vi "Move to End.vi"   [LabVIEW 2017, in "Drivers.lvlib" / "ASI TG-1000.lvlib"]
uses:
  ASI TG-1000.lvlib
  Public/Utility/Axis Name.ctl
types:
  T1 = typedef "Drivers.lvlib/ASI TG-1000.lvlib/Axis Name.ctl" = enum8{"undefined", "A", "B", "C", "D", "E", "F", "G", "H", "I", "J", "K", "L", "M", "N", "O", "P", "Q", "R", "S", "T", "U", "V", "W", "X", "Y", "Z"}
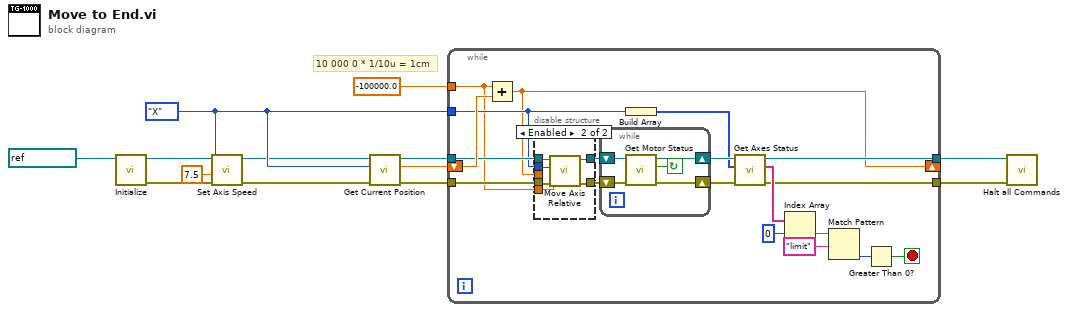
[diagram p0: block diagram]
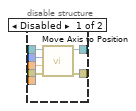
[diagram p2: hidden frame]
diagram:
  w5 = Axis_Name."X" ("Axis")
  # "10 000 0 * 1/10u = 1cm"
  n1 = call "Initialize.vi"("VISA resource name"=refnum<visa-resource-name> "COM13") -> ("error out"=w12:errorcluster, "VISA resource name out"=w11:refnum<visa-resource-name>)  [unwired: 9 in]
  n2 = call "Set Axis Speed.vi"("error in (no error)"=w12, "Speed (mm/s)"=7.5, "Axis"=w5, "VISA resource name"=w11) -> ("error out"=w1:errorcluster, "VISA out"=w2:refnum<visa-resource-name>)  [unwired: 6 in]
  n3 = call "Get Current Position.vi"("error in (no error)"=w1, "Axis"=w5, "VISA in"=w2) -> ("error out"=w9:errorcluster, "position [internal units]"=w8:dbl, "VISA out"=w6:refnum<visa-resource-name>)  [unwired: 6 in]
  n4 = while {
    tunnel: w9 -> [w30]
    shift-right: [w15] -> _
    shift-left: w8 -> [w29]
    tunnel: -100000.0 ("Position [internal units]") -> [w14]
    tunnel: w6 -> [w28]
    tunnel: w5 -> [w25]
    tunnel: [w19] -> w3
    tunnel: [w16] -> w4
    stop <- w17 stop-if-true
    n5 = Add(x=w14, y=w29) -> (x+y=w15:dbl)
    n6 = disable-structure shown="Enabled" {
      disable-tunnel: [w38 w42] -> w32
      disable-tunnel: [w37 w43] -> w31
      disable-tunnel: w30 -> [w36 w44]
      disable-tunnel: w28 -> [w35 w41]
      disable-tunnel: w25 -> [w34 w40]
      disable-tunnel: w15 -> [w33 _]
      disable-tunnel: w14 -> [_ w39]
      frame Disabled {
        n7 = call "Move Axis to Position.vi"("error in (no error)"=w36, "Position [internal units]"=w33, "Axis"=w34, "VISA in"=w35) -> ("error out"=w37:errorcluster, "VISA out"=w38:refnum<visa-resource-name>)  [unwired: 5 in]
      }
      frame Enabled {
        n8 = call "Move Axis Relative.vi"("error in (no error)"=w44, "Relative Position [internal units]"=w39, "Axis"=w40, "VISA in"=w41) -> ("error out"=w43:errorcluster, "VISA out"=w42:refnum<visa-resource-name>)  [unwired: 5 in]
      }
    }
    n9 = while {
      shift-right: [w46] -> w26
      shift-left: w31 -> [w49]
      shift-right: [w47] -> w27
      shift-left: w32 -> [w48]
      stop <- w45 continue-if-true
      n10 = call "Get Motor Status.vi"("error in (no error)"=w49, "VISA in"=w48) -> ("error out"=w46:errorcluster, "Motors Busy?"=w45:bool, "VISA out"=w47:refnum<visa-resource-name>)  [unwired: 6 in]
    }
    n11 = Build Array(w25) -> (w24:T1[])
    n12 = call "Get Axes Status.vi"("error in (no error)"=w26, "Array of axes"=w24, "VISA in"=w27) -> ("error out"=w19:errorcluster, "Array of status strings"=w23:string[], "VISA out"=w16:refnum<visa-resource-name>)  [unwired: 6 in]
    n13 = Index Array(array=w23, index=0) -> (element=w21:string)
    n14 = Match Pattern(string=w21, regular expression="limit") -> (offset past match=w18:i32)  [unwired: 1 in, 3 out]
    n15 = Greater Than 0?(x=w18) -> (x > 0?=w17:bool)
  }
  n16 = call "Halt all Commands.vi"("error in (no error)"=w3, "VISA in"=w4) -> ()  [unwired: 7 in, 2 out]
